vi "Byte Buffer.Set pointers.vi"(8 "error in (no error)":errorcluster, 10 "Byte Buffer pointers":T1, 11 "Byte Buffer in":refnum<class "Byte Buffer.lvclass">) -> (0 "error out":errorcluster, 3 "Byte Buffer out":refnum<class "Byte Buffer.lvclass">)   [LabVIEW 2016, in "VeriStand Data.lvlib" / "Byte Buffer.lvclass"]
uses:
  Byte Buffer.lvclass
  Byte Buffer.Pointers.ctl
  Byte Buffer.lvclass/Byte Buffer.ctl
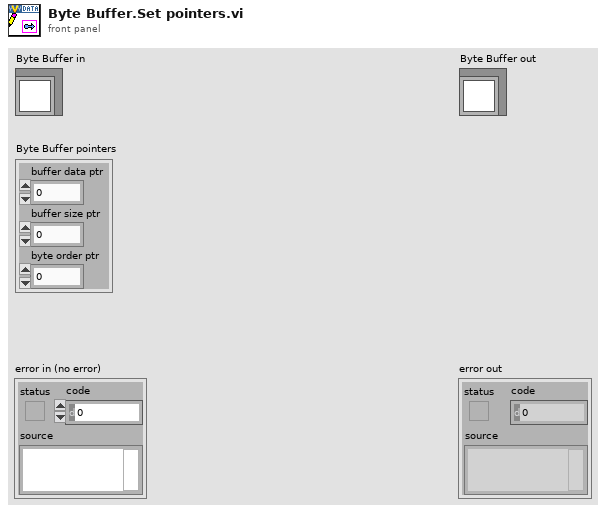
[diagram p1: front panel]
types:
  T1 = typedef "VeriStand Data.lvlib/Byte Buffer.lvclass/Byte Buffer.Pointers.ctl" = cluster{"buffer data ptr":u64, "buffer size ptr":u64, "byte order ptr":u64}
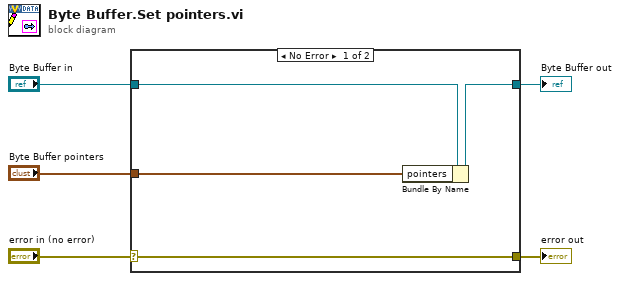
[diagram p0: block diagram]
diagram:
  n1 = case shown="No Error" "error in (no error)" {
    selector: "error in (no error)" -> [w9 w10]
    tunnel: [w9 w10] -> w4
    tunnel: [w7 w11] -> w2
    tunnel: "Byte Buffer in" -> [w8 w11]
    tunnel: "Byte Buffer pointers" -> [w6 _]
    frame No Error {
      n2 = Bundle By Name(cluster=w8, "pointers"=w6) -> (w7:refnum<class "Byte Buffer.lvclass">)
    }
    frame Error {
    }
  }
  "error out" <- w4
  "Byte Buffer out" <- w2
